vi "Extended Image To Frames.vi"(11 "Extended Image":T2) -> (2 "Delays":i32[](array[numeric]), 3 "Frames":T1[](array[typedef]))   [LabVIEW 2020, in "G-Image.lvlib"]
doc: "Convert the extended image type to one or more frames. Use with animated GIF data."
uses:
  G-Image.lvlib
  Extended Image.ctl
  <vilib>/picture/picture.llb/imagedata.ctl
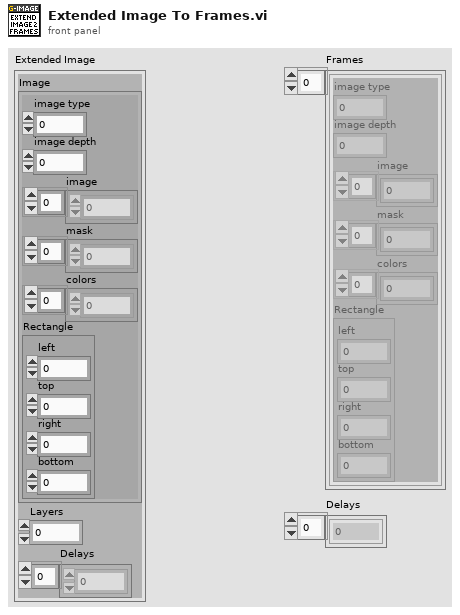
[diagram p1: front panel]
types:
  T1 = typedef "imagedata.ctl" = cluster{"image type":i32, "image depth":i32, "image":u8[], "mask":u8[], "colors":u32[], "Rectangle":cluster{"left":i16, "top":i16, "right":i16, "bottom":i16}}
  T2 = typedef "G-Image.lvlib/Extended Image.ctl" = cluster{"Image":T1, "Layers":i32, "Delays":i32[]}
  T3 = cluster{"left":i16, "top":i16, "right":i16, "bottom":i16}
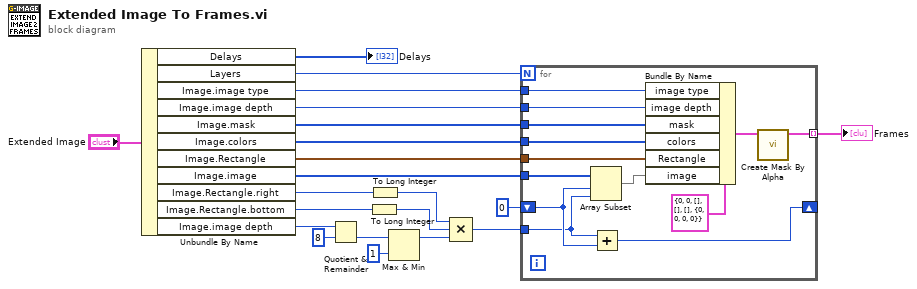
[diagram p0: block diagram]
diagram:
  n1 = Unbundle By Name("Extended Image") -> ("Delays"=→"Delays":i32[], "Layers"=w20:i32, "Image.image type"=w5:i32, "Image.image depth"=w4:i32, "Image.mask"=w3:u8[], "Image.colors"=w2:u32[], "Image.Rectangle"=w1:T3, "Image.image"=w19:u8[], "Image.Rectangle.right"=w18:i16, "Image.Rectangle.bottom"=w17:i16, "Image.image depth"=w14:i32)
  n2 = Quotient & Remainder(x=w14, y=8) -> (floor(x/y)=w12:i32)  [unwired: 1 out]
  n3 = To Long Integer(number=w17) -> (32bit integer=w15:i32)
  n4 = To Long Integer(number=w18) -> (32bit integer=w16:i32)
  n5 = Max & Min(x=w12, y=1) -> (max(x,y)=w10:i32)  [unwired: 1 out]
  n6 = Compound Arithmetic op=MULTIPLY(w16, w15, w10) -> (w8:i32)
  n7 = for {
    N: w20 -> [_]
    tunnel: w19 -> [w34]
    tunnel: w8 -> [w32]
    shift-right: [w31] -> _
    shift-left: 0 -> [w33]
    tunnel: w1 -> [w22]
    tunnel: [w28] -> w6 mode=indexing
    tunnel: w5 -> [w26]
    tunnel: w4 -> [w25]
    tunnel: w3 -> [w24]
    tunnel: w2 -> [w23]
    n8 = Array Subset(array=w34, index=w33, length=w32) -> (w30:u8[])
    n9 = Add(x=w32, y=w33) -> (x+y=w31:i32)
    n10 = Bundle By Name(cluster=T1 {"image type"=0, "image depth"=0, "image"=[], "mask"=[], "colors"=[], "Rectangle"={"left"=0, "top"=0, "right"=0, "bottom"=0}} ("masked image data"), "image type"=w26, "image depth"=w25, "mask"=w24, "colors"=w23, "Rectangle"=w22, "image"=w30) -> (w29:T1)
    n11 = call <vilib>:"Create Mask By Alpha.vi"("image data"=w29) -> ("masked image data"=w28:T1)  [unwired: 10 in]
  }
  "Frames" <- w6
